vi "Chebybezier1.vi"(9 "order":u32=3, 10 "end":dbl=1.0 format="%.2f", 11 "start":dbl format="%.2f") -> (2 "x/y":dbl, 3 "X values":dbl[][](array[numeric]))   [LabVIEW 2019]
panel:
  out "error":i32
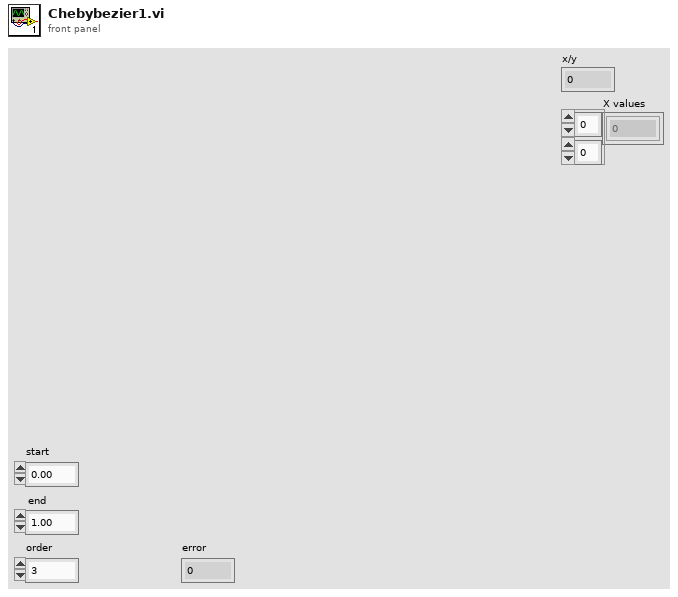
[diagram p1: front panel]
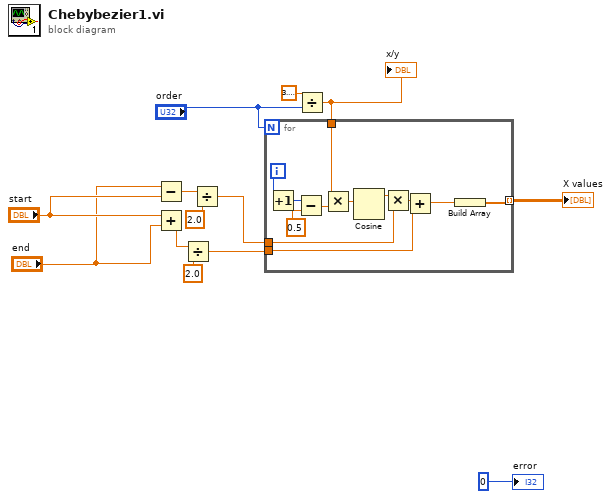
[diagram p0: block diagram]
diagram:
  n1 = Subtract(x="end", y="start") -> (x-y=w9:dbl)
  n2 = Add(x="start", y="end") -> (x+y=w11:dbl)
  n3 = Divide(x=w11, y=2.0) -> (x/y=w2:dbl)
  n4 = Divide(x=w9, y=2.0) -> (x/y=w3:dbl)
  n5 = Divide(x=3.141592653589793, y="order") -> (x/y=w5:dbl)
  "x/y" <- w5
  n6 = for {
    N: "order" -> [_]
    tunnel: w5 -> [w23]
    tunnel: w3 -> [w19]
    tunnel: w2 -> [w16]
    tunnel: [w14] -> w1 mode=indexing
    i -> [w24]
    n7 = Increment(x=w24) -> (x+1=w20:i32)
    n8 = Subtract(x=w20, y=0.5) -> (x-y=w22:dbl)
    n9 = Multiply(x=w23, y=w22) -> (x*y=w21:dbl)
    n10 = Cosine(x=w21) -> (cos(x)=w18:dbl)
    n11 = Multiply(x=w18, y=w19) -> (x*y=w17:dbl)
    n12 = Add(x=w17, y=w16) -> (x+y=w15:dbl)
    n13 = Build Array(w15) -> (w14:dbl[])
  }
  "X values" <- w1
  "error" <- 0
